vi "SailSetSuggestions-OLD.vi"() -> ()   [LabVIEW 2013]
doc: "Returns suggestions for the sail positions (0-1) based on the current state of the boat. This outputs a number of suggestions, which are blended in the arbiter in Act.\n\nInputs: relative wind angle, degree of luffing, rudder force, the direction of the boat, and the desired direction of the boat.\n\nAngles should follow the Sailbot standard of 0 East and CCW increase, except for Relative Wind. Velocities should be in (m/s). RudderForce and DegreeOfLuffing are not settled yet, but 0-1 would be reasonable.\n\nEric Schneider and Bonnie Ishiguro, Jan. 2014"
uses:
  Data/TypeDefs/Sail Set Suggestions.ctl
  Data/TypeDefs/Rudder Set Suggestions.ctl
  Data/TypeDefs/MB Think to Act Bundled Sail Commands.ctl
panel:
  in  "Current Main Position":dbl
  in  "Current Jib Position":dbl
  in  "DesiredProportionOfBoatSpeed (01)":dbl
  out "SailSuggestionToMB-ACTArbiter":T1 {"GetOutOfIronsSailSuggestion"."MainSailSuggestion" min=0.0 max=1.0; "GetOutOfIronsSailSuggestion"."JibSailSuggestion" min=0.0 max=1.0; "GetOutOfIronsRudder" min=-1.0 max=1.0; "SailByWindLookup"."MainSailSuggestion" min=0.0 max=1.0; "SailByWindLookup"."JibSailSuggestion" min=0.0 max=1.0; "SailsByTurningBoat"."MainSailSuggestion" min=0.0 max=1.0; "SailsByTurningBoat"."JibSailSuggestion" min=0.0 max=1.0; "SailByTurtleMode"."MainSailSuggestion" min=0.0 max=1.0; "SailByTurtleMode"."JibSailSuggestion" min=0.0 max=1.0; "RudderByTurtleMode" min=-1.0 max=1.0; "SailsByReducingLuffing"."MainSailSuggestion" min=0.0 max=1.0; "SailsByReducingLuffing"."JibSailSuggestion" min=0.0 max=1.0; "SailsByBalancingRudder"."MainSailSuggestion" min=0.0 max=1.0; "SailsByBalancingRudder"."JibSailSuggestion" min=0.0 max=1.0; "TackManeuverSails"."MainSailSuggestion" min=0.0 max=1.0; "TackManeuverSails"."JibSailSuggestion" min=0.0 max=1.0; "TackManeuverRudder" min=-1.0 max=1.0; "JibeManeuverSails"."MainSailSuggestion" min=0.0 max=1.0; "JibeManeuverSails"."JibSailSuggestion" min=0.0 max=1.0; "JibeManeuverRudder" min=-1.0 max=1.0}
  in  "BoatSpeed (m/s)":dbl
  in  "WindSpeed (m/s)":dbl
  in  "AbsoluteWindAngle (0-360)":dbl
  in  "DesiredHeading (0-360)":dbl
  in  "RobotHeading (0-360)":dbl
  in  "RudderForce":dbl
  in  "DegreeOfLuffing (0-1)?":dbl
  in  "RelativeWindAngle (0-180)":dbl
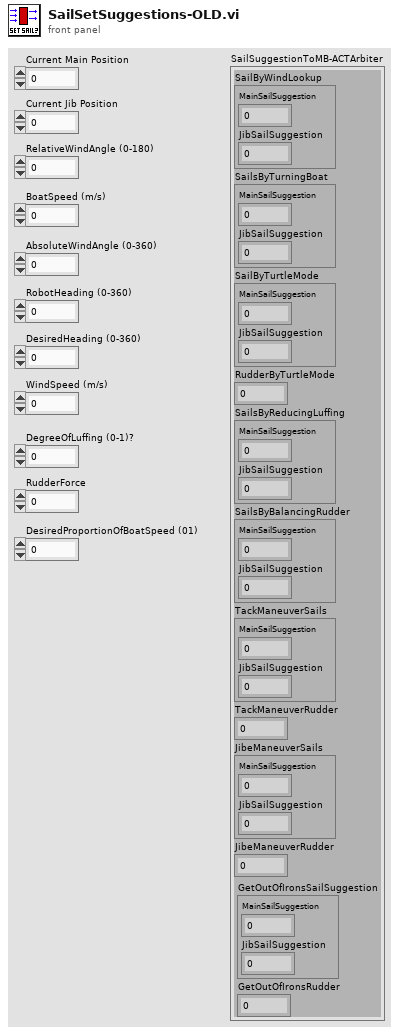
[diagram p1: front panel]
types:
  T1 = typedef "MB Think to Act Bundled Sail Commands.ctl" = cluster{"SailByWindLookup":T2, "SailsByTurningBoat":T2, "SailByTurtleMode":T2, "RudderByTurtleMode":T3, "SailsByReducingLuffing":T2, "SailsByBalancingRudder":T2, "TackManeuverSails":T2, "TackManeuverRudder":T3, "JibeManeuverSails":T2, "JibeManeuverRudder":T3, "GetOutOfIronsRudder":T3, "GetOutOfIronsSailSuggestion":T2}
  T2 = typedef "Sail Set Suggestions.ctl" = cluster{"MainSailSuggestion":dbl, "JibSailSuggestion":dbl}
  T3 = typedef "Rudder Set Suggestions.ctl" = dbl
  T4 = cluster{"BoatVelocityInY":dbl, "BoatVelocityInX":dbl}
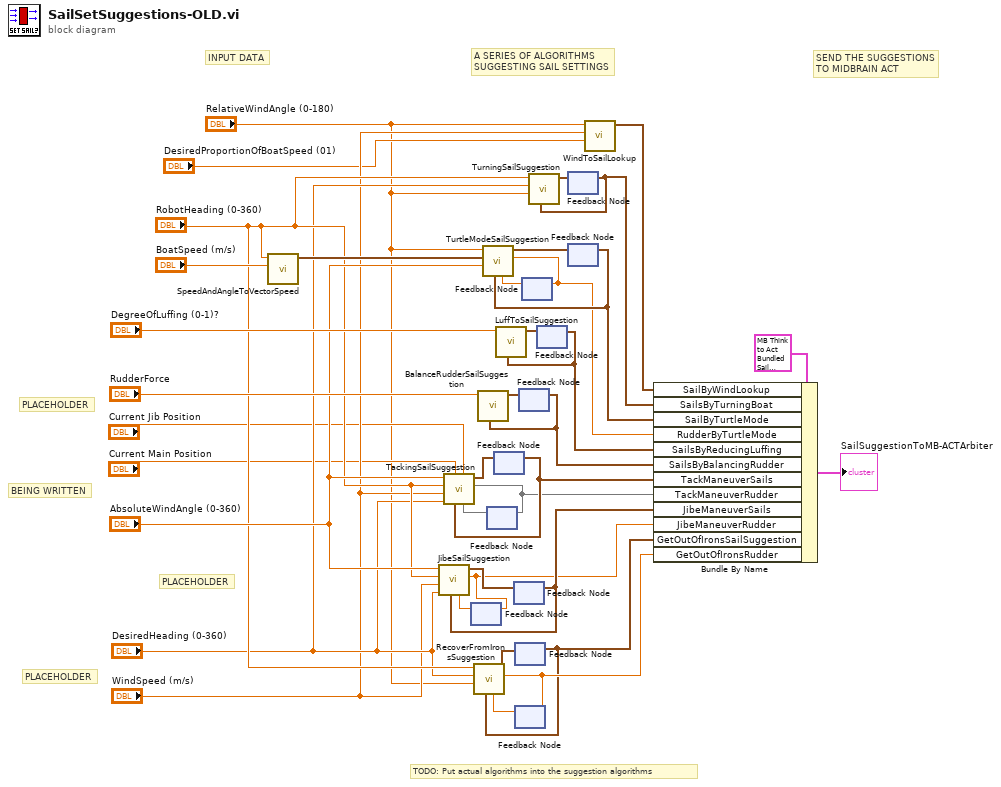
[diagram p0: block diagram]
diagram:
  # "PLACEHOLDER"
  # "BEING WRITTEN"
  # "PLACEHOLDER"
  # "PLACEHOLDER"
  # "SEND THE SUGGESTIONS\nTO MIDBRAIN ACT"
  # "A SERIES OF ALGORITHMS\nSUGGESTING SAIL SETTINGS"
  # "INPUT DATA"
  # "TODO: Put actual algorithms into the suggestion algorithms"
  n1 = call "SpeedAndAngleToVectorSpeed.vi"("BoatSpeed (m/s)"="BoatSpeed (m/s)", "RobotHeading (deg)"="RobotHeading (0-360)") -> ("BoatVectorVelocity"=w16:T4)  [unwired: 9 in]
  n2 = feedback #1() -> (w30:T3)  [unwired: 1 in]
  n3 = feedback #2() -> (w28)  [unwired: 1 in]
  n4 = feedback #3() -> (w21:T2)  [unwired: 1 in]
  n5 = call "TackingSailSuggestion.vi"(4:w28, 5:"Current Jib Position", 6:w21, 7:"Current Main Position", "RobotHeading"="DesiredHeading (0-360)", "DesiredHeading"="WindSpeed (m/s)", "ApparentWindAngle"="RobotHeading (0-360)", "AbsoluteWindAngle"="AbsoluteWindAngle (0-360)") -> (2:w17, "Suggested Sail Setpoints"=w29:T2)  [unwired: 2 in]
  n6 = feedback-in #2(w17) -> ()
  n7 = feedback-in #3(w29) -> ()
  n8 = feedback #4() -> (w20:T2)  [unwired: 1 in]
  n9 = call "JibeSailSuggestion.vi"("OLD Suggested Rudder Setpoint"=w30, "OLD Suggested Sail Setpoints"=w20, "DesiredHeading"="DesiredHeading (0-360)", "WindSpeed"="WindSpeed (m/s)", "RobotHeading"="RobotHeading (0-360)", "AbsoluteWindAngle"="AbsoluteWindAngle (0-360)") -> ("Suggested Rudder Setpoint"=w12:T3, "Suggested Sail Setpoints"=w31:T2)  [unwired: 4 in]
  n10 = feedback-in #1(w12) -> ()
  n11 = feedback-in #4(w31) -> ()
  n12 = feedback #5() -> (w6:T2)  [unwired: 1 in]
  n13 = feedback #6() -> (w8:dbl)  [unwired: 1 in]
  n14 = call "RecoverFromIronsSuggestion.vi"("Old Rudder"=w8, "Old Suggested Sail Setpoints"=w6, "RelativeWindAngle"="RelativeWindAngle (0-180)", "DesiredHeading"="DesiredHeading (0-360)", "RobotHeading"="RobotHeading (0-360)") -> ("Suggested Rudder Set Point"=w9:dbl, "Suggested Sail Setpoints"=w7:T2)  [unwired: 5 in]
  n15 = feedback-in #5(w7) -> ()
  n16 = feedback-in #6(w9) -> ()
  n17 = feedback #7() -> (w18:T2)  [unwired: 1 in]
  n18 = call "BalanceRudderSailSuggestion.vi"("OLD Suggested Sail Setpoints"=w18, "ForceOnRudder"="RudderForce") -> ("Suggested Sail Setpoints"=w26:T2)  [unwired: 9 in]
  n19 = feedback-in #7(w26) -> ()
  n20 = feedback #8() -> (w32:T3)  [unwired: 1 in]
  n21 = feedback #9() -> (w19:T2)  [unwired: 1 in]
  n22 = call "LuffToSailSuggestion.vi"("OLD Suggested Sail Setpoints"=w19, "DegreeOfLuffing"="DegreeOfLuffing (0-1)?") -> ("Suggested Sail Setpoints"=w27:T2)  [unwired: 9 in]
  n23 = feedback-in #9(w27) -> ()
  n24 = feedback #10() -> (w24:T2)  [unwired: 1 in]
  n25 = call "TurningSailSuggestion.vi"("Old Suggested Sail Setpoints"=w24, "RelativeWindAngle"="RelativeWindAngle (0-180)", "DesiredHeading"="DesiredHeading (0-360)", "RobotHeading"="RobotHeading (0-360)") -> ("Suggested Sail Setpoints"=w34:T2)  [unwired: 7 in]
  n26 = feedback-in #10(w34) -> ()
  n27 = feedback #11() -> (w23:T2)  [unwired: 1 in]
  n28 = call "TurtleModeSailSuggestion.vi"("OLD Suggested Rudder Setpoint"=w32, "OLD Suggested Sail Setpoints"=w23, "AbsoluteWindAngle"="AbsoluteWindAngle (0-360)", "BoatVectorVelocity"=w16, "RelativeWindAngle"="RelativeWindAngle (0-180)") -> ("Suggested Rudder Setpoint"=w22:T3, "Suggested Sail Setpoints"=w33:T2)  [unwired: 5 in]
  n29 = feedback-in #8(w22) -> ()
  n30 = feedback-in #11(w33) -> ()
  n31 = call "WindToSailLookup.vi"("DesiredProportionOfBoatSpeed"="DesiredProportionOfBoatSpeed (01)", "WindSpeed"="WindSpeed (m/s)", "ApparentWindAngle"="RelativeWindAngle (0-180)") -> ("Suggested Sail Setpoints"=w25:T2)  [unwired: 8 in]
  n32 = Bundle By Name(cluster=T1 {"SailByWindLookup"={"MainSailSuggestion"=0.0, "JibSailSuggestion"=0.0}, "SailsByTurningBoat"={"MainSailSuggestion"=0.0, "JibSailSuggestion"=0.0}, "SailByTurtleMode"={"MainSailSuggestion"=0.0, "JibSailSuggestion"=0.0}, "RudderByTurtleMode"=0.0, "SailsByReducingLuffing"={"MainSailSuggestion"=0.0, "JibSailSuggestion"=0.0}, "SailsByBalancingRudder"={"MainSailSuggestion"=0.0, "JibSailSuggestion"=0.0}, "TackManeuverSails"={"MainSailSuggestion"=0.0, "JibSailSuggestion"=0.0}, "TackManeuverRudder"=0.0, "JibeManeuverSails"={"MainSailSuggestion"=0.0, "JibSailSuggestion"=0.0}, "JibeManeuverRudder"=0.0, "GetOutOfIronsRudder"=0.0, "GetOutOfIronsSailSuggestion"={"MainSailSuggestion"=0.0, "JibSailSuggestion"=0.0}} ("SailSuggestionToMB-ACTArbiter"), "SailByWindLookup"=w25, "SailsByTurningBoat"=w24, "SailByTurtleMode"=w23, "RudderByTurtleMode"=w22, "SailsByReducingLuffing"=w19, "SailsByBalancingRudder"=w18, "TackManeuverSails"=w21, "TackManeuverRudder"=w17, "JibeManeuverSails"=w20, "JibeManeuverRudder"=w12, "GetOutOfIronsSailSuggestion"=w6, "GetOutOfIronsRudder"=w9) -> (→"SailSuggestionToMB-ACTArbiter":T1)
